vi "parse -- get list of matches -- numbers.vi"(10 "regexp":string="([\\d\\.\\+\\-]+)\\,?\\s*", 11 "string":string="c11, c22, c33, c23, c13, c12, c44, c55,  c66") -> (0 "Array of strings":string[](array[string])=["c11", "c22", "c33", "c23", "c13", "c12", "c44", "c55", "c66"], 1 "# of numbers":i32=9, 2 "after match":string, 3 "Array of numbers":dbl[](array[numeric]))   [LabVIEW 2015]
uses:
  <vilib>/regexp/Match Regular Expression.xnode
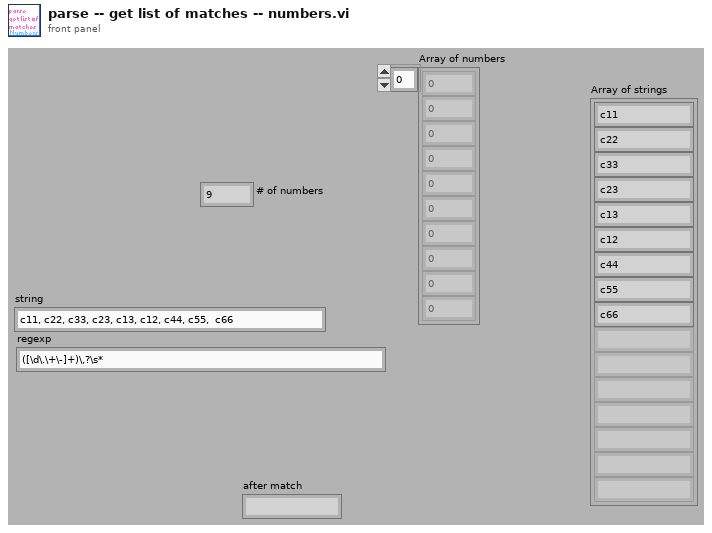
[diagram p1: front panel]
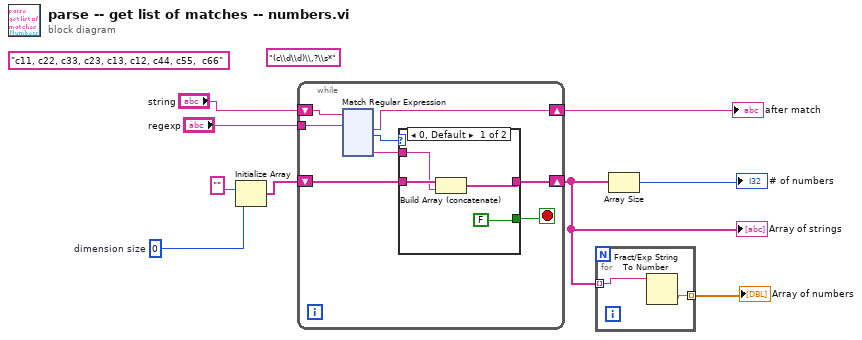
[diagram p0: block diagram]
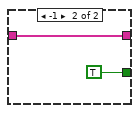
[diagram p2: hidden frame]
diagram:
  w4 = 0  # dimension size
  (unwired) "c11, c22, c33, c23, c13, c12, c44, c55,  c66" ("format string")
  (unwired) "(c\\d\\d)\\,?\\s*" ("format string")
  n1 = Initialize Array("" ("format string"), w4) -> (w3:string[])
  n2 = while {
    tunnel: "regexp" -> [w17]
    shift-right: [w16] -> w8
    shift-left: "string" -> [w15]
    shift-right: [w12] -> w1
    shift-left: w3 -> [w11]
    stop <- w13 stop-if-true
    n3 = xnode "Match Regular Expression"("input string"=w15, "regular expression"=w17) -> ("after match"=w16:string, "offset past match"=w14:i32, "submatch 1"=w10:string)  [unwired: 4 in, 3 out]
    n4 = case shown="0, Default" w14 {
      tunnel: [FALSE TRUE] -> w13
      tunnel: [w18 w22] -> w12
      tunnel: w11 -> [w20 w22]
      tunnel: w10 -> [w19 _]
      frame 0, Default {
        n5 = Build Array (concatenate)(w20, w19) -> (w18:string[])
      }
      frame -1 {
      }
    }
  }
  "after match" <- w8
  "Array of strings" <- w1
  n6 = for {
    tunnel: w1 -> [w141] mode=indexing
    tunnel: [w140] -> w2 mode=indexing
    n7 = Fract/Exp String To Number(string=w141) -> (number=w140:dbl)  [unwired: 3 in, 1 out]
  }
  "Array of numbers" <- w2
  n8 = Array Size(array=w1) -> (size(s)=→"# of numbers":i32)
